vi "Real time state machine - Saccade suppression LED.vi"() -> ()   [LabVIEW 2013]
uses:
  <vilib>/Platform/TimedLoop/XDataNode/timing_clust.ctl
  <vilib>/Platform/TimedLoop/XDataNode/nitl_modes.ctl
  <vilib>/Platform/TimedLoop/XDataNode/wakeup.ctl
  <vilib>/DAQmx/write.llb/DAQmx Write (Digital 1D Bool NChan 1Samp 1Line).vi
  <vilib>/DAQmx/read.llb/DAQmx Read (Analog 1D DBL NChan 1Samp).vi
  <vilib>/DAQmx/write.llb/DAQmx Write (Analog DBL 1Chan 1Samp).vi
  <vilib>/platform/TimedLoop/XDataNode/XDataNode.xnode
  <vilib>/Platform/TimedLoop/XDataNode/XDNodeRunTimeDep.lvlib
panel:
  out "x degree out":dbl
  in  "Saccade min degrees per 3 frames":dbl=5.0
  in  "Saccade max degrees per 3 frames":dbl=15.0
  out "Min":dbl
  out "Sec":dbl=47.16078567504883
  in  "Display length (S)":sgl=10.0
  out "shaft encoder":waveform(sgl)(graph)={"t0"=timestamp(3524542772.3366966 s since 1904-01-01), "dt"=0.02, "Y"=array[500 elements]}
  out "Current state":T1(ring)=enum."VS"
  out "# of rewards":i32
  in  "Automatic reward":bool=TRUE
  out "Lick reward":bool
  out "RT FIFO (DISP)":u32(slide) scale=0.0..50.0
  out "RT FIFO (Log)":u32(slide) scale=0.0..50.0
  out "Digital Waveform Graph":digitalwaveform(graph)={"t0"=timestamp(3524542772.3366966 s since 1904-01-01), "dt"=0.0004, "Y"={"transitions"=[], "data"=array25000x3[75000 elements]}, "error"={"status"=FALSE, "code"=37421928, "source"=""}}
  out "Trial # (State machine)":u32=1
  out "Actual cycle period (uS)":i64=94
  in  "State machine cycle (uS)":i64=200
  in  "Save file to":string="C:\\ni-rt\\LabVIEW Data\\"
  in  "RT FIFO size":u32=50
  in  "VS filter period (uS)":i32=500
  out "Start one trial":bool
  out "Trial Done":bool
  out "error out":errorcluster
  out "Busy":bool
  out "Trial #":i32=1
  out "Save data":bool
  out "LED?":bool
  out "Pulse amp 0":sgl
  out "Pulse amp 1":sgl
  out "Pulse delay":sgl
  out "Pulse width":sgl
  out "Pulse period (ms)":sgl
  out "Pulse #":sgl
  out "Reward period (uS)":u32
  out "Reward start delay (uS)":u32
  out "Water duration (uS)":u32=30000
  out "Water refractory period (uS)":u32=500000
  out "Shock duration (uS)":u32=10000
  out "Shock refractory period (uS)":u32=1000000
  out "Trial timeout (uS)":u32=3000000
  out "Lick threshold (V)":fxp<+,32,16>=1.600006103515625
  out "Track eye":bool=TRUE
  out "Allow shock":bool
  out "Allow timeout":bool
  out "Manually give water":bool
  out "Manually give shock":bool
  out "VS threshold (V)":fxp<+,32,16>=0.5
  out "VS type":string="continuous_flash"
  out "File name":string="Test"
  out "Behavior type":string="fullfield"
  in  "Stop state":bool
  in  "Remote port":u16=9090
  in  "Remote IP_Main":string="192.168.137.10"
  in  "Local port":u16=9091
  in  "Local IP_This computer":string="192.168.137.2"
  out "ABORT":bool
  out "Initial data received":bool
  # "VS"
  # "Behavior"
  # "Trial #"
  # "Received parameters"
  # "Time to wait for reward window"
  # "Elapsed time"
  # "Min"
  # "Sec"
  # "Controls"
  # "Network"
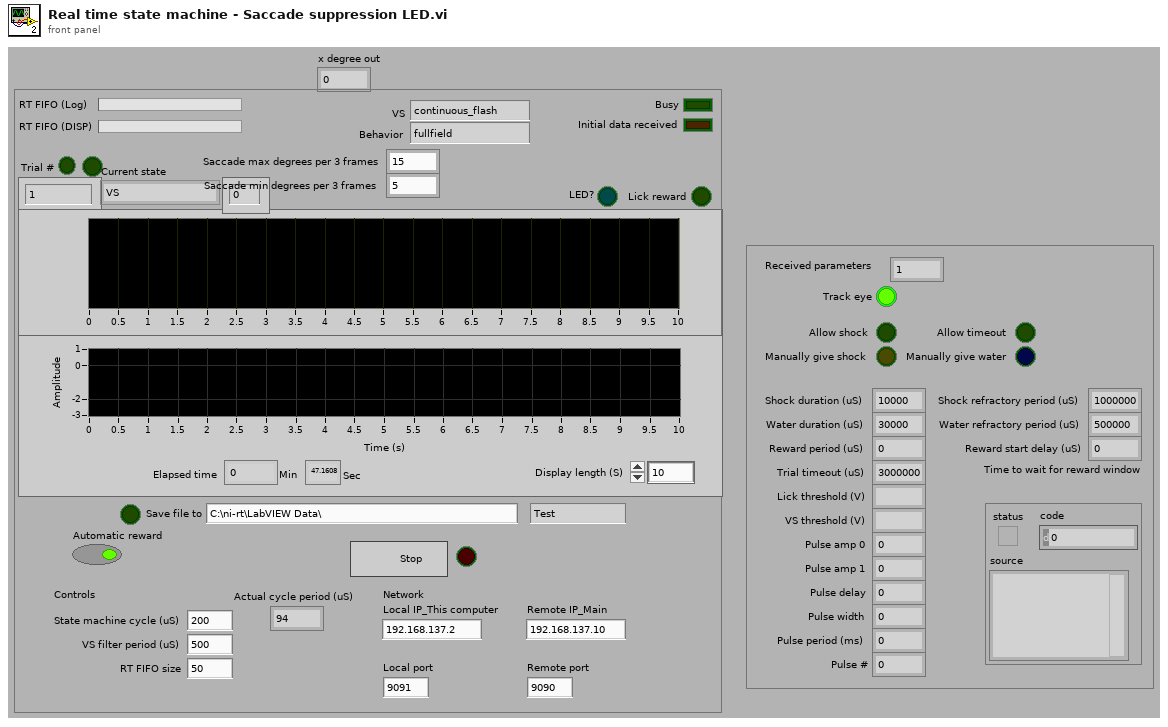
[diagram p1: front panel]
types:
  T1 = enum16{"Idle", "Before VS", "VS", "VS2", "After VS", "Wait for lever press", "Cycle End", "Reward", "Reward Refractory", "Punish", "Punish Refractory", "Exit", "Timeout", "Lick reward"}
  T2 = enum16{"open", "replace", "create", "open or create", "replace or create", "replace or create with confirmation"}
  T3 = typedef "XDNodeRunTimeDep.lvlib/timing_clust.ctl" = cluster{"Expected End [f-1]":u64, "Actual End [f-1]":u64, "Finished Late? [f-1]":bool, "Expected End [i-1]":u64, "Actual End [i-1]":u64, "Finished Late? [i-1]":bool, "Expected Start [i]":u64, "Actual Start [i]":u64, "Expected Start [f]":u64, "Actual Start [f]":u64, "Source Name":string, "Structure Name":string, "Period":i64, "Deadline":i64, "Offset":i64, "Start":i64, "Priority":i32, "Timeout":i32, "Mode":T4, "Wakeup Reason":T5, "Error":errorcluster, "Source Type":string, "Secondary Source Type":string, "Global End Time":u64, "Global Start Time":u64, "Frame Duration":u64, "Iteration Duration":u64, "Assigned CPU":i32, "I/O Scan Engine Mode":u32}
  T4 = typedef "XDNodeRunTimeDep.lvlib/nitl_modes.ctl" = enum32{"No Change", "Process missed periods, maintain original phase", "Discard missed periods, maintain original phase", "Process missed periods, ignore original phase", "Discard missed periods, ignore original phase"}
  T5 = typedef "XDNodeRunTimeDep.lvlib/wakeup.ctl" = enum32{"Normal", "Aborted", "Asynchronous wakeup", "Timing source error", "Timed loop error", "Timeout"}
  T6 = enum16{"big-endian, network order", "native, host order", "little-endian"}
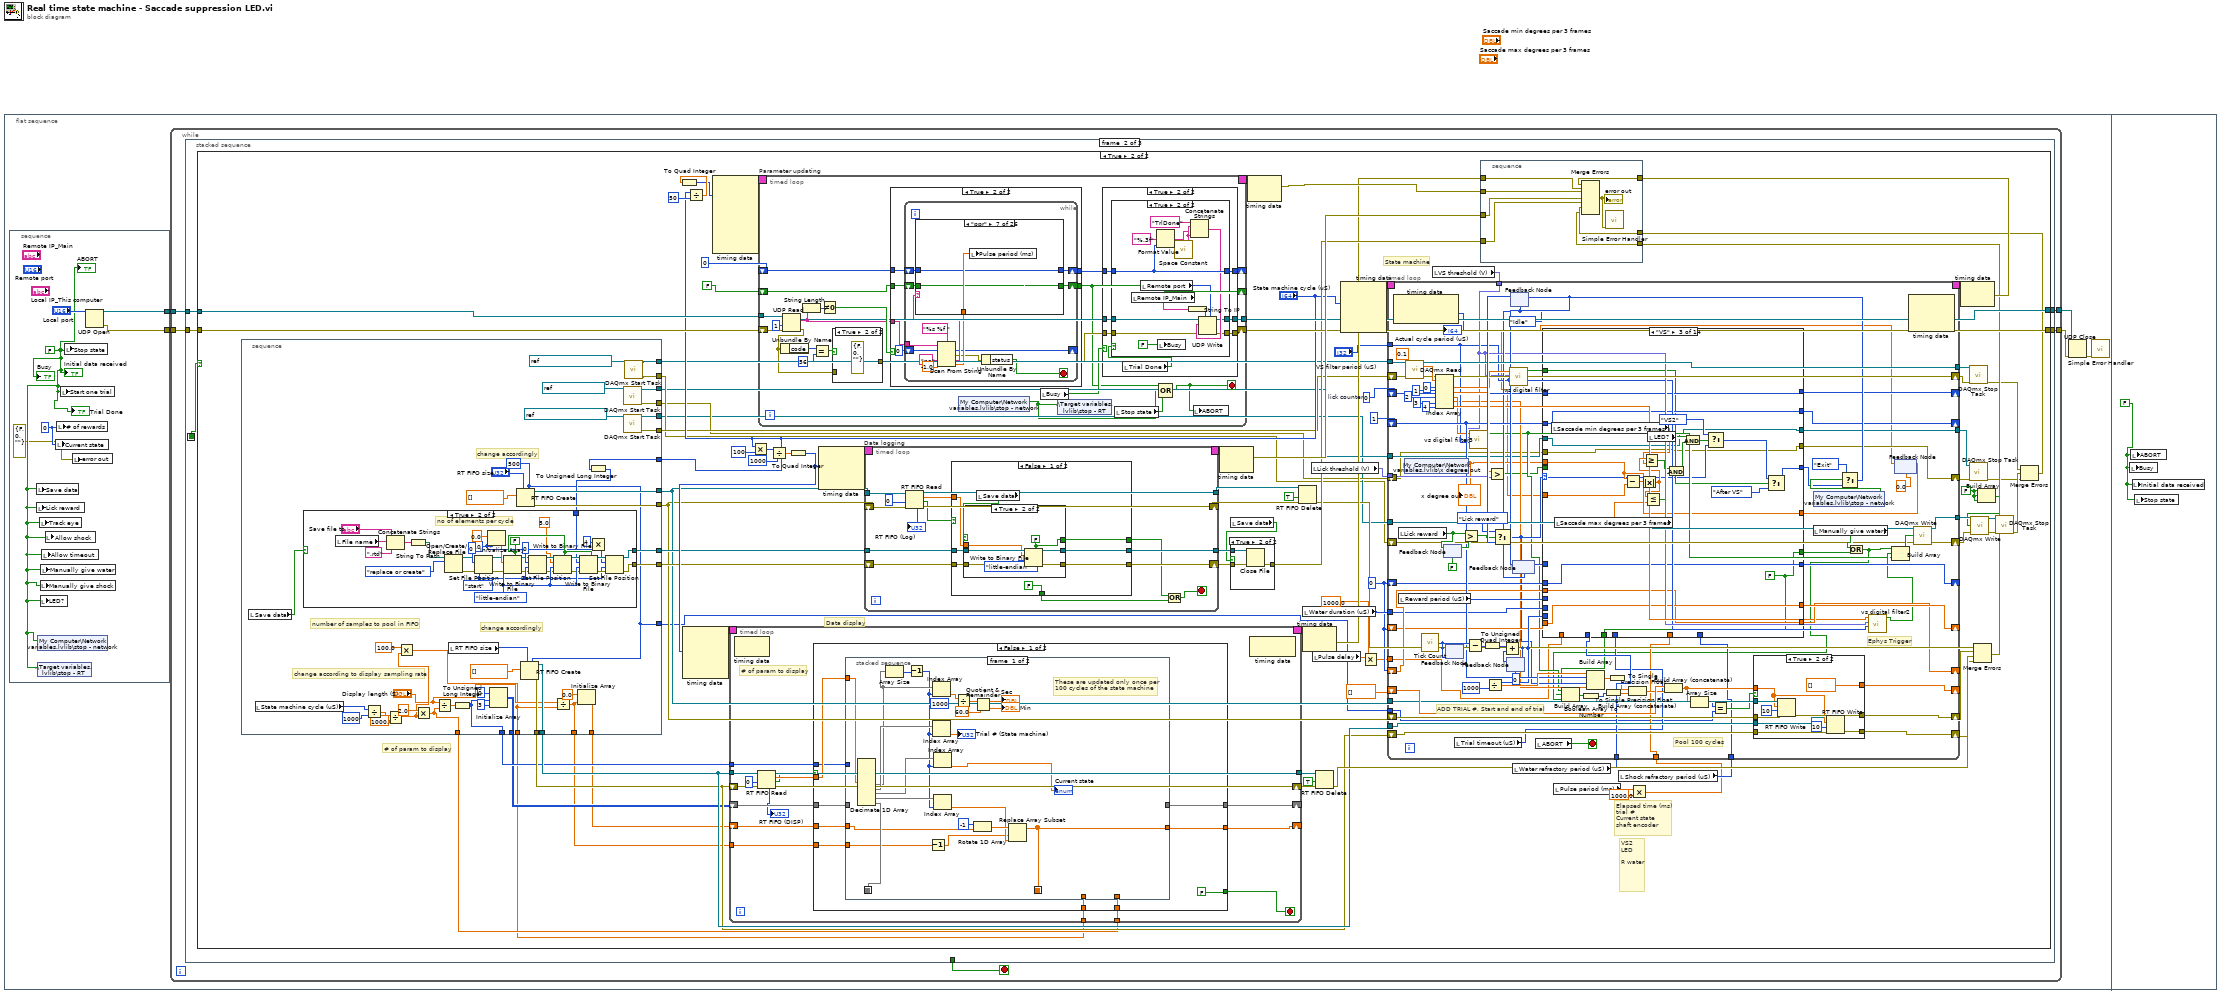
[diagram p0: block diagram]
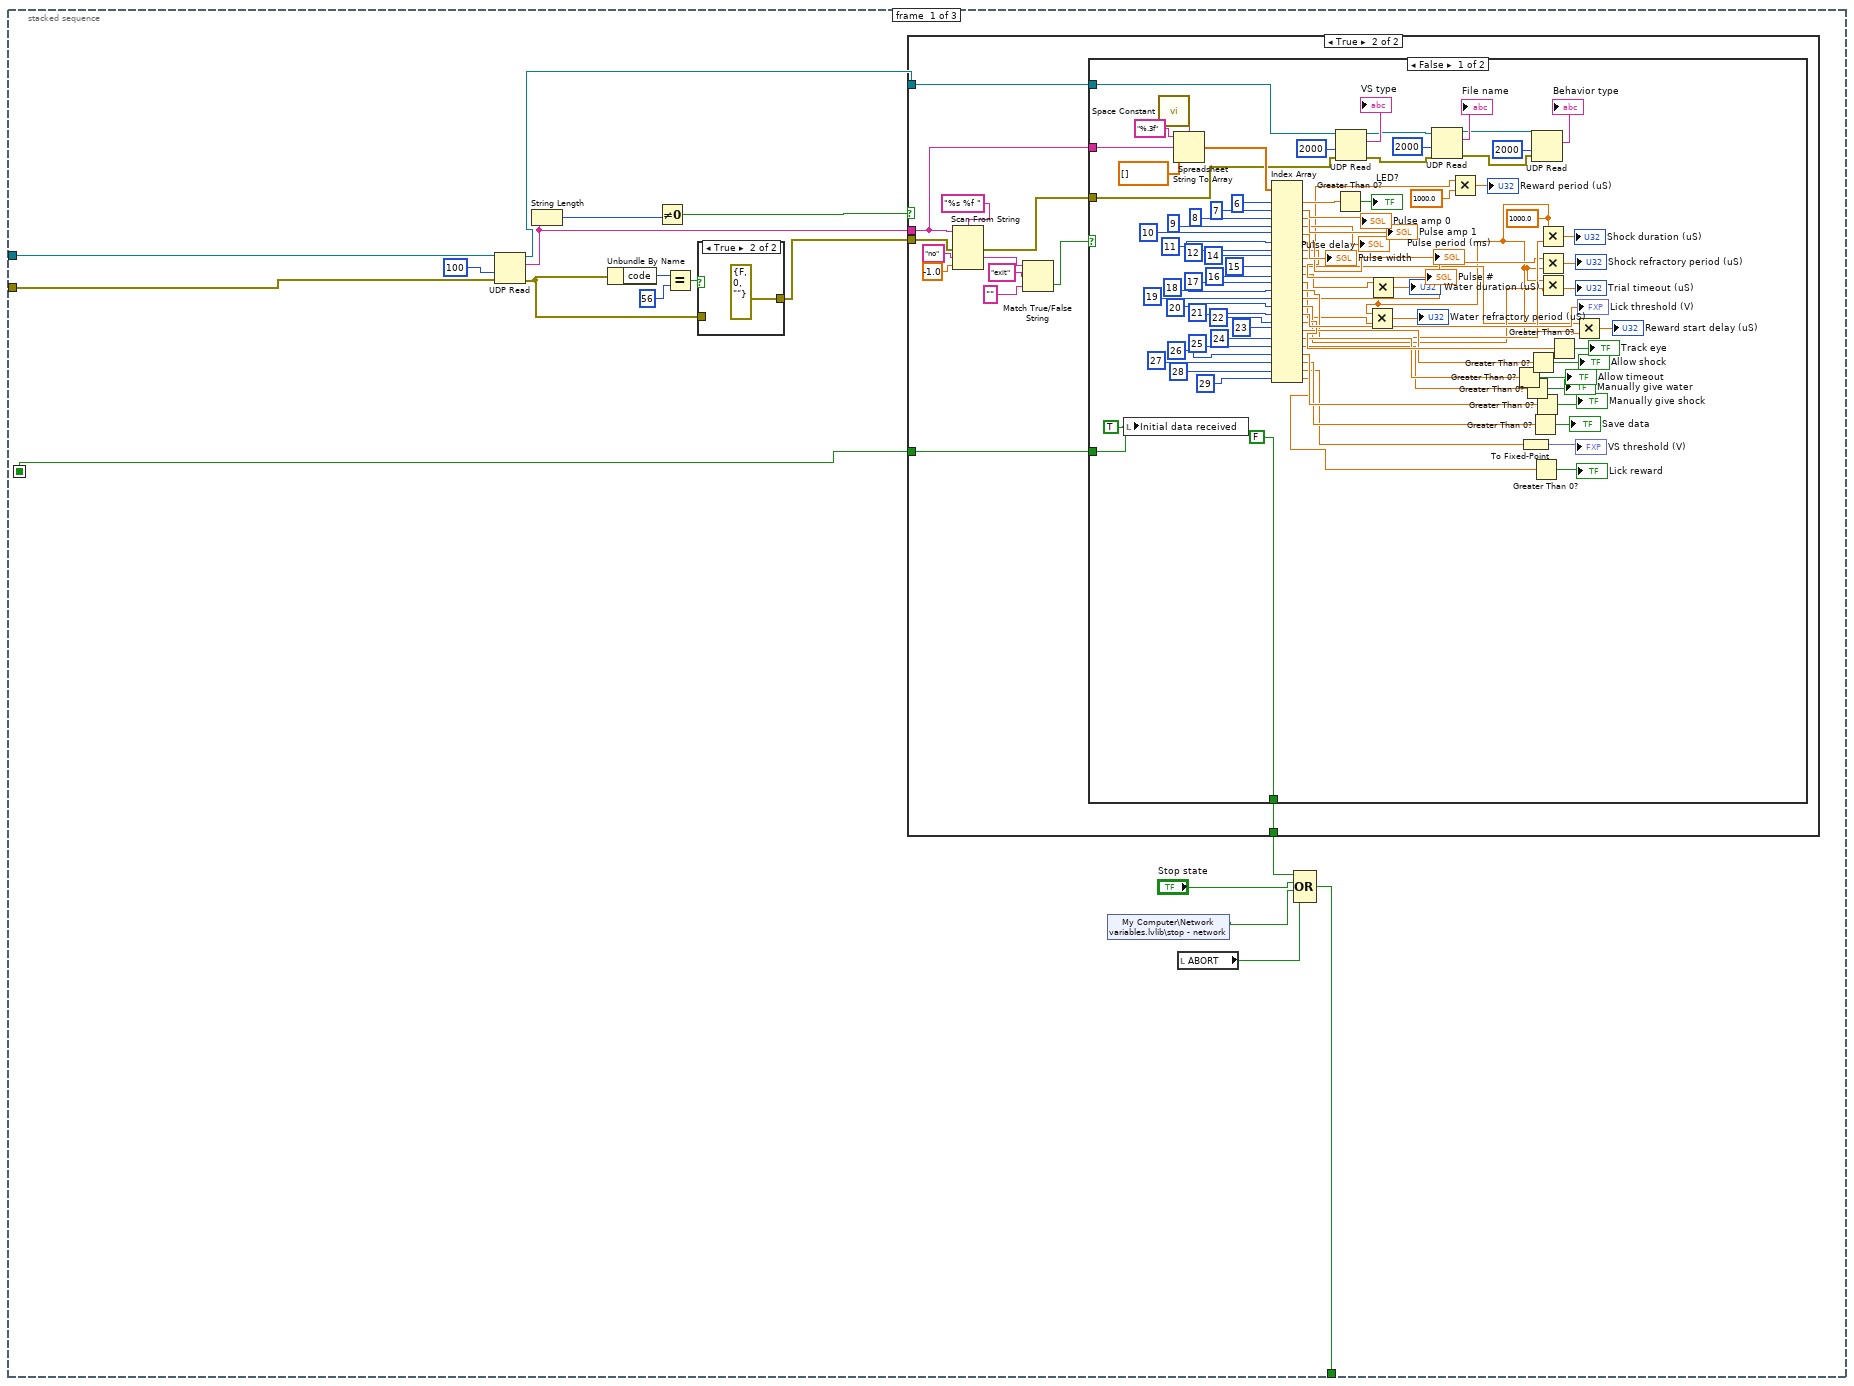
[diagram p2: hidden frame]
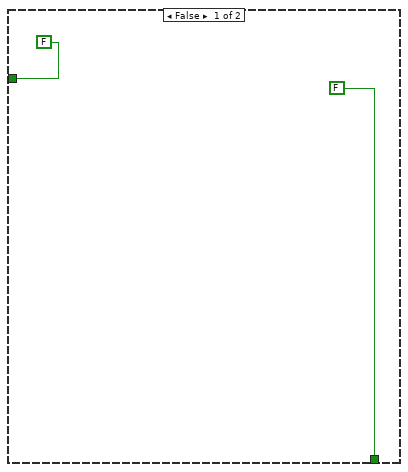
[diagram p3: hidden frame]
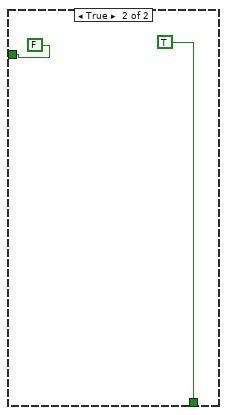
[diagram p4: hidden frame]
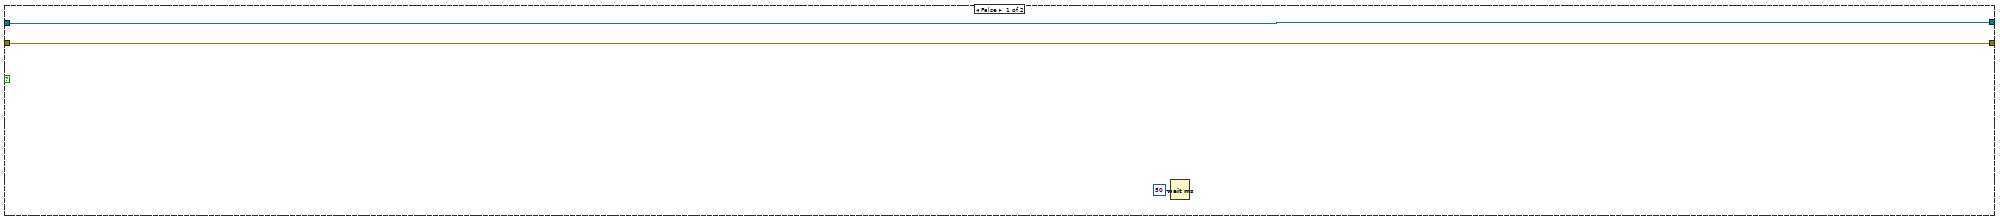
[diagram p6: hidden frame]
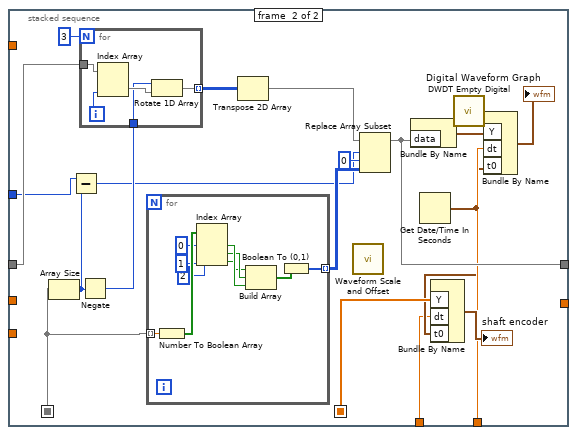
[diagram p9: hidden frame]
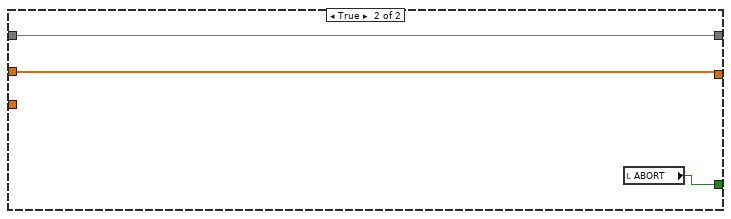
[diagram p10: hidden frame]
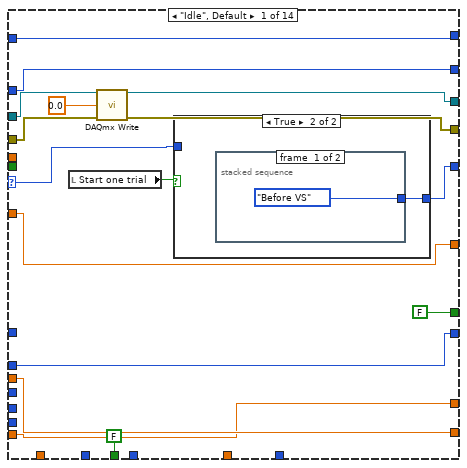
[diagram p11: hidden frame]
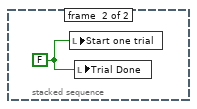
[diagram p13: hidden frame]
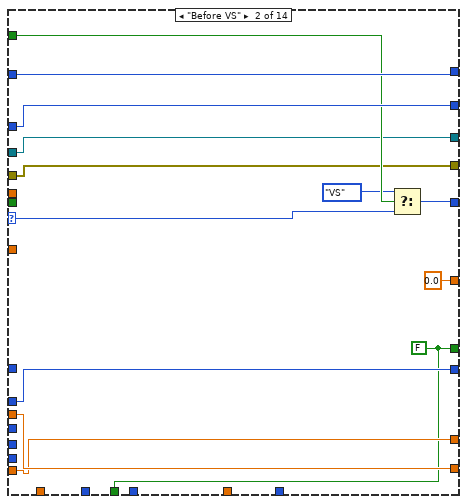
[diagram p14: hidden frame]
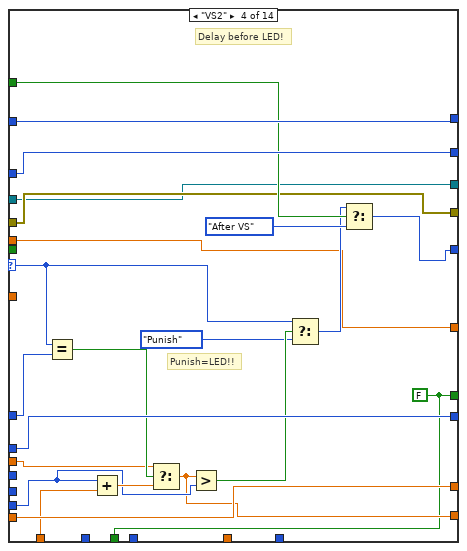
[diagram p15: hidden frame]
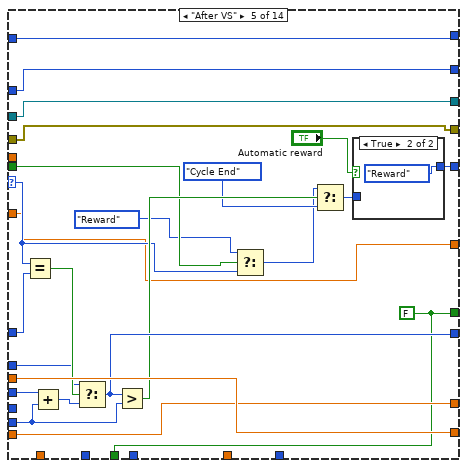
[diagram p16: hidden frame]
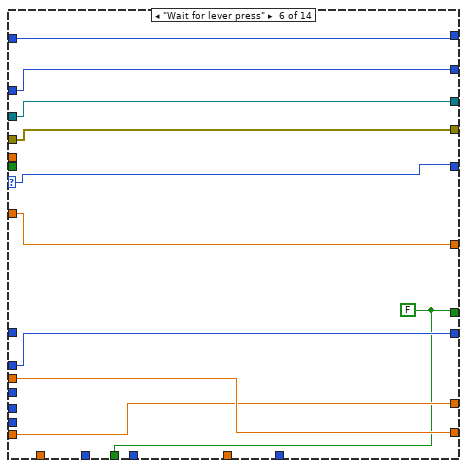
[diagram p18: hidden frame]
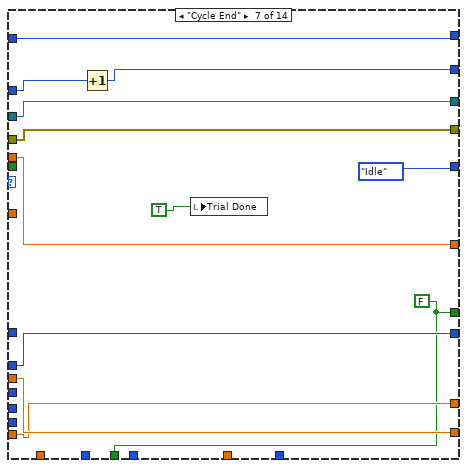
[diagram p19: hidden frame]
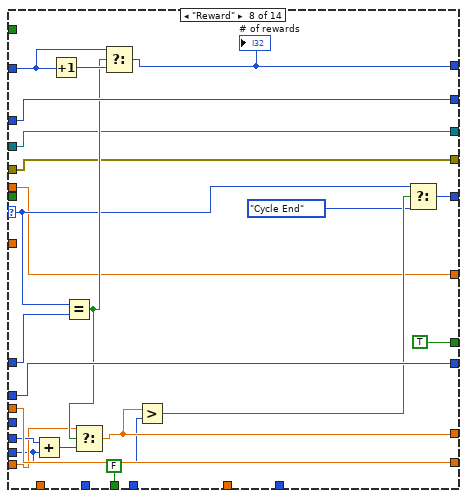
[diagram p20: hidden frame]
diagram:
  n1 = flat-sequence {
    frame #0 {
      n2 = stacked-sequence {
        tunnel: [w1027] -> w5
        tunnel: [w1026] -> w4
        frame #0 {
          w1025 = 0
          w1024 = FALSE
          n3 = local write "Save data"(w1024) -> ()
          n4 = local write "Lick reward"(w1024) -> ()
          n5 = shared-variable "My Computer\\Network variables.lvlib\\stop - network"(w1024) -> ()  [unwired: 1 in, 1 out]
          n6 = shared-variable ".\\Target variables.lvlib\\stop - RT"(w1024) -> ()  [unwired: 1 in, 1 out]
          n7 = local write "Track eye"(w1024) -> ()
          n8 = local write "Manually give shock"(w1024) -> ()
          n9 = local write "LED?"(w1024) -> ()
          n10 = local write "Manually give water"(w1024) -> ()
          n11 = local write "Allow timeout"(w1024) -> ()
          n12 = local write "Allow shock"(w1024) -> ()
          n13 = local write "Current state"(w1025) -> ()
          n14 = local write "# of rewards"(w1025) -> ()
          n15 = local write "Start one trial"(w1024) -> ()
          n16 = local write "Stop state"(w1024) -> ()
          n17 = local write "error out"(errorcluster {"status"=FALSE, "code"=0, "source"=""} ("error out")) -> ()
          n18 = UDP Open(11:"Local port") -> (port=w1027:refnum<k16>, 0:w1026:errorcluster)  [unwired: 4 in, 1 out]
          "ABORT" <- w1024
          "Initial data received" <- w1024
          "Busy" <- w1024
          "Trial Done" <- w1024
        }
      }
      n19 = while {
        tunnel: w5 -> [w10]
        tunnel: w4 -> [w9]
        tunnel: [w8] -> w3
        tunnel: [w7] -> w2
        stop <- w6 stop-if-true
        n20 = stacked-sequence {
          seq-local: [w16 _ _] -> [_ w135 _]
          tunnel: w10 -> [w27 w132 _]
          tunnel: w9 -> [w26 w133 _]
          tunnel: [w15 _ _] -> w6
          tunnel: [_ w134 _] -> w8
          tunnel: [_ w131 _] -> w7
          frame #0 {
            n21 = UDP Read(connection ID=w27, timeout ms (25000)=100, 8:w26) -> (data out=w18:string, error out=w22:errorcluster, 3:w17:refnum<k16>)  [unwired: 1 in, 2 out]
            n22 = String Length(string=w18) -> (length=w21:i32)
            n23 = Unbundle By Name(w22) -> ("code"=w25:i32)
            n24 = Not Equal To 0?(x=w21) -> (x != 0?=w20:bool)
            n25 = Equal?(x=w25, y=56) -> (x = y?=w23:bool)
            n26 = case shown="True" w23 {
              tunnel: w22 -> [w129 _]
              tunnel: [w129 errorcluster {"status"=FALSE, "code"=0, "source"=""} ("error out")] -> w19
              frame False {
              }
              frame True {
              }
            }
            n27 = case shown="True" w20 {
              tunnel: w19 -> [_ w41]
              tunnel: w18 -> [_ w35]
              tunnel: w17 -> [_ w33]
              tunnel: [FALSE w32] -> w14
              tunnel: [FALSE w31] -> w16
              frame False {
              }
              frame True {
                n28 = Scan From String(format string="%s %f ", input string=w35, error in=w41, default 1="no" ("default value 1"), default 2=sgl -1.0 ("default value 1")) -> (error out=w34:errorcluster, output 1=w39:string)  [unwired: 2 in, 2 out]
                n29 = Match True/False String(2:"" ("false string"), 3:"exit" ("true string"), 4:w39) -> (0:w36:bool)  [unwired: 1 out]
                n30 = case shown="False" w36 {
                  tunnel: w35 -> [w123 _]
                  tunnel: w34 -> [w81 _]
                  tunnel: w33 -> [w80 _]
                  tunnel: [FALSE TRUE] -> w32
                  tunnel: [w68 FALSE] -> w31
                  frame False {
                    w49 = sgl 1000.0
                    w68 = TRUE
                    n31 = local write "Initial data received"(w68) -> ()
                    n32 = call <vilib>:"Space Constant.vi"() -> ("String"=w125:string)
                    n33 = Spreadsheet String To Array(delimiter (Tab)=w125, format string="%.3f", spreadsheet string=w123, array type (2D Dbl)=sgl[] []) -> (array=w122:sgl[])
                    n34 = Index Array(array=w122, index #1=6 ("index"), index #2=7 ("index"), index #3=8 ("index"), index #4=9 ("index"), index #5=10 ("index"), index #6=11 ("index"), index #7=12 ("index"), index #8=14 ("index"), index #9=15 ("index"), index #10=16 ("index"), index #11=17 ("index"), index #12=18 ("index"), index #13=19 ("index"), index #14=20 ("index"), index #15=21 ("index"), index #16=22 ("index"), index #17=23 ("index"), index #18=24 ("index"), index #19=25 ("index"), index #20=26 ("index"), index #21=27 ("index"), index #22=28 ("index"), index #23=29 ("index")) -> (element #1=w120:sgl, element #2=→"Pulse amp 0":sgl, element #3=→"Pulse amp 1":sgl, element #4=→"Pulse delay":sgl, element #5=→"Pulse width":sgl, element #6=→"Pulse period (ms)":sgl, element #7=→"Pulse #":sgl, element #8=w64:sgl, element #9=w55:sgl, element #10=w53:sgl, element #11=w51:sgl, element #12=w61:sgl, element #13=w60:sgl, element #14=w57:sgl, element #15=→"Lick threshold (V)":sgl, element #16=w94:sgl, element #17=w91:sgl, element #18=w89:sgl, element #19=w86:sgl, element #20=w84:sgl, element #21=w46:sgl, element #22=w45:sgl, element #23=w44:sgl)
                    n35 = Greater Than 0?(x=w120) -> (x > 0?=→"LED?":bool)
                    n36 = UDP Read(connection ID=w80, timeout ms (25000)=2000, 8:w81) -> (data out=→"VS type":string, error out=w76:errorcluster, 3:w74:refnum<k16>)  [unwired: 1 in, 2 out]
                    n37 = Multiply(x=w49, y=w51) -> (x*y=→"Water refractory period (uS)":sgl)
                    n38 = Multiply(x=w53, y=w49) -> (x*y=→"Water duration (uS)":sgl)
                    n39 = UDP Read(connection ID=w74, timeout ms (25000)=2000, 8:w76) -> (data out=→"File name":string, error out=w72:errorcluster, 3:w71:refnum<k16>)  [unwired: 1 in, 2 out]
                    n40 = Multiply(x=w64, y=sgl 1000.0) -> (x*y=→"Reward period (uS)":sgl)
                    n41 = Greater Than 0?(x=w89) -> (x > 0?=→"Allow timeout":bool)
                    n42 = To Fixed-Point(number=w45) -> (fixed-point=→"VS threshold (V)":fxp<+/-,32,16>)  [unwired: 1 in]
                    n43 = Greater Than 0?(x=w86) -> (x > 0?=→"Manually give water":bool)
                    n44 = Greater Than 0?(x=w91) -> (x > 0?=→"Allow shock":bool)
                    n45 = Greater Than 0?(x=w46) -> (x > 0?=→"Save data":bool)
                    n46 = Greater Than 0?(x=w44) -> (x > 0?=→"Lick reward":bool)
                    n47 = UDP Read(connection ID=w71, timeout ms (25000)=2000, 8:w72) -> (data out=→"Behavior type":string)  [unwired: 1 in, 4 out]
                    n48 = Greater Than 0?(x=w84) -> (x > 0?=→"Manually give shock":bool)
                    n49 = Multiply(x=w49, y=w61) -> (x*y=→"Shock duration (uS)":sgl)
                    n50 = Multiply(x=w60, y=w49) -> (x*y=→"Shock refractory period (uS)":sgl)
                    n51 = Multiply(x=w49, y=w57) -> (x*y=→"Trial timeout (uS)":sgl)
                    n52 = Greater Than 0?(x=w94) -> (x > 0?=→"Track eye":bool)
                    n53 = Multiply(x=w55, y=w49) -> (x*y=→"Reward start delay (uS)":sgl)
                  }
                  frame True {
                  }
                }
              }
            }
            n54 = shared-variable "My Computer\\Network variables.lvlib\\stop - network"() -> (w11:bool)  [unwired: 1 in, 1 out]
            n55 = local read "ABORT"() -> (w12:bool)
            n56 = Compound Arithmetic op=OR(w14, "Stop state", w11, w12) -> (w15:bool)
          }
          frame #1 {
            n57 = case shown="True" w135 {
              tunnel: w133 -> [w138 w221]
              tunnel: [w138 w213] -> w134
              tunnel: w132 -> [w137 w220]
              tunnel: [w137 w212] -> w131
              frame False {
                n58 = Wait (ms)(milliseconds to wait=u32 50) -> ()  [unwired: 1 out]
              }
              frame True {
                w165 = FALSE
                w201 = 0  # lick counter
                w158 = 0
                # "VS2\nLED\n\nR water"
                # "# of param to display"
                # "Data display"
                # "Elapsed time (ms)\ntrial #\nCurrent state\nshaft encoder"
                # "State machine"
                n59 = stacked-sequence {
                  tunnel: [w273] -> w186
                  tunnel: [w272] -> w185
                  tunnel: [w269] -> w184
                  tunnel: [w268] -> w183
                  tunnel: [w254] -> w166
                  tunnel: [w249] -> w182
                  tunnel: [w260] -> w181
                  tunnel: "State machine cycle (uS)" -> [w253]
                  tunnel: [w257] -> w179
                  tunnel: [w256] -> w178
                  tunnel: [w251] -> w157
                  tunnel: [w248] -> w156
                  tunnel: [w244] -> w155
                  tunnel: [w243] -> w154
                  tunnel: [w241] -> w144
                  tunnel: [w240] -> w143
                  tunnel: [w238] -> w142
                  tunnel: [w237] -> w141
                  tunnel: [w235] -> w140
                  tunnel: [w234] -> w139
                  frame #0 {
                    w251 = u32 500 ("elements in array (1)")
                    # "number of samples to pool in FIFO"
                    # "change according to display sampling rate"
                    # "change accordingly"
                    # "change accordingly"
                    n60 = local read "Save data"() -> (w274:bool)
                    n61 = local read "State machine cycle (uS)"() -> (w261:i64)
                    n62 = Divide(x=w261, y=u32 1000) -> (x/y=w263:dbl)
                    n63 = Divide(x=w263, y=1000.0) -> (x/y=w246:dbl)
                    n64 = Multiply(x=100.0, y=w246) -> (x*y=w244:dbl)
                    n65 = Multiply(x=2.0, y=w246) -> (x*y=w254:dbl)
                    n66 = Divide(x="Display length (S)", y=w254) -> (x/y=w266:dbl)
                    n67 = local read "RT FIFO size"() -> (w271:u32)
                    n68 = To Unsigned Long Integer(number=w266) -> (unsigned 32bit integer=w249:u32)
                    n69 = Initialize Array(u8 0 ("element"), w249, 3 ("dimension size")) -> (w260:u8[][])
                    n70 = RT FIFO Create(1:sgl[] [], 4:"RT FIFO size", 6:w251) -> (8:w257:refnum<k33>, 11:w256:errorcluster)  [unwired: 5 in, 1 out]
                    n71 = RT FIFO Create(1:sgl[] [], 4:w271, 6:w251) -> (8:w269:refnum<k33>, 11:w268:errorcluster)  [unwired: 5 in, 1 out]
                    n72 = Divide(x="Display length (S)", y=w244) -> (x/y=w243:dbl)
                    n73 = Initialize Array(sgl 0.0 ("element"), w243) -> (w248:sgl[])
                    n74 = To Unsigned Long Integer(number=w253) -> (unsigned 32bit integer=w252:u32)
                    n75 = case shown="True" w274 {
                      tunnel: [_ w278] -> w273
                      tunnel: [_ w277] -> w272
                      tunnel: w252 -> [_ w276]
                      frame False {
                      }
                      frame True {
                        w299 = FALSE
                        w292 = 10 ("dimension size")
                        w300 = T6."little-endian" ("byte order (0:big-endian, network order)")
                        w291 = enum16{"start", "end", "current"}."start" ("from (0:start)")
                        # "no of elements per cycle"
                        n76 = local read "File name"() -> (w302:string)
                        n77 = Concatenate Strings("Save file to", w302, ".rtd" ("string")) -> (w305:string)
                        n78 = String To Path(string=w305) -> (path=w306:path)
                        n79 = Open/Create/Replace File(file path (use dialog)=w306, operation (0:open)=T2."replace or create") -> (refnum out=w279:refnum<file>, error out=w280:errorcluster)  [unwired: 4 in, 1 out]
                        n80 = Set File Position(offset (in bytes) (0)=i64 0, refnum=w279, from (0:start)=w291, error in=w280) -> (refnum out=w282:refnum<file>, error out=w283:errorcluster)
                        n81 = Initialize Array(sgl 0.0 ("element"), w292) -> (w285:sgl[])
                        n82 = Write to Binary File(file (use dialog)=w282, data=w285, error in=w283, 5:w299, 9:w300) -> (refnum out=w287:refnum<file>, error out=w286:errorcluster)  [unwired: 1 in, 1 out]
                        n83 = Set File Position(offset (in bytes) (0)=i64 0, refnum=w287, from (0:start)=w291, error in=w286) -> (refnum out=w289:refnum<file>, error out=w290:errorcluster)
                        n84 = Write to Binary File(file (use dialog)=w289, data=sgl 5.0, error in=w290, 5:w299, 9:w300) -> (refnum out=w297:refnum<file>, error out=w295:errorcluster)  [unwired: 1 in, 1 out]
                        n85 = Write to Binary File(file (use dialog)=w297, data=w276, error in=w295, 5:w299, 9:w300) -> (refnum out=w298:refnum<file>, error out=w296:errorcluster)  [unwired: 1 in, 1 out]
                        n86 = Multiply(x=4, y=w292) -> (x*y=w294:i32)
                        n87 = Set File Position(offset (in bytes) (0)=w294, refnum=w298, from (0:start)=w291, error in=w296) -> (refnum out=w277:refnum<file>, error out=w278:errorcluster)
                      }
                    }
                    n88 = call <vilib>:"DAQmx Start Task.vi"("task/channels in"=refnum<k21> "LED analog out" ("DAQmx Task Name")) -> ("task out"=w238:refnum<k21>, "error out"=w237:errorcluster)  [unwired: 13 in]
                    n89 = call <vilib>:"DAQmx Start Task.vi"("task/channels in"=refnum<k21> "Digital_write_saccade" ("DAQmx Task Name")) -> ("task out"=w235:refnum<k21>, "error out"=w234:errorcluster)  [unwired: 13 in]
                    n90 = call <vilib>:"DAQmx Start Task.vi"("task/channels in"=refnum<k21> "Analog_read_saccade" ("DAQmx Task Name")) -> ("task out"=w241:refnum<k21>, "error out"=w240:errorcluster)  [unwired: 13 in]
                  }
                }
                n91 = Divide(x="State machine cycle (uS)", y=i64 50) -> (x/y=w191:dbl)
                n92 = To Quad Integer(1:w191) -> (0:w190:i64)
                n93 = node-c288 ("Input Node")(w190) -> (w229:T3)  [unwired: 6 in]
                n94 = Multiply(x="State machine cycle (uS)", y=u32 100) -> (x*y=w194:i64)
                n95 = timed-loop "Parameter updating" {
                  timing: w229 -> [_]
                  timing-out: [_] -> w228
                  tunnel: w220 -> [w860]
                  shift-right: [w845] -> w213
                  shift-left: w221 -> [w861]
                  shift-right: [w848] -> _
                  shift-left: 0 -> [w851]
                  tunnel: [w844] -> w212
                  shift-right: [w842] -> _
                  shift-left: FALSE -> [w852]
                  stop <- w843 stop-if-true
                  n96 = UDP Read(connection ID=w860, timeout ms (25000)=1, 8:w861) -> (data out=w853:string, error out=w856:errorcluster, 3:w846:refnum<k16>)  [unwired: 1 in, 2 out]
                  n97 = Unbundle By Name(w856) -> ("code"=w859:i32)
                  n98 = String Length(string=w853) -> (length=w855:i32)
                  n99 = Equal?(x=w859, y=56) -> (x = y?=w857:bool)
                  n100 = Not Equal To 0?(x=w855) -> (x != 0?=w854:bool)
                  n101 = case shown="True" w857 {
                    tunnel: w856 -> [w1013 _]
                    tunnel: [w1013 errorcluster {"status"=FALSE, "code"=0, "source"=""} ("error out")] -> w847
                    frame False {
                    }
                    frame True {
                    }
                  }
                  n102 = case shown="True" w854 {
                    tunnel: w853 -> [_ w896]
                    tunnel: w852 -> [w889 w895]
                    tunnel: w851 -> [w890 w894]
                    tunnel: [w890 w893] -> w849
                    tunnel: [w889 w892] -> w842
                    frame False {
                    }
                    frame True {
                      n103 = while {
                        tunnel: w896 -> [w908]
                        shift-right: [w904] -> w892
                        shift-left: w895 -> [w905]
                        shift-right: [w903] -> w893
                        shift-left: w894 -> [w902]
                        shift-right: [w898] -> _
                        shift-left: u32 0 -> [w899]
                        stop <- w900 stop-if-true
                        n104 = Scan From String(format string="%s %f ", input string=w908, initial scan location=w899, default 1="no" ("default value 1"), default 2=-1.0 ("default value 2")) -> (offset past scan=w898:u32, error out=w901:errorcluster, output 1=w907:string, output 2=w906:dbl)  [unwired: 1 in, 1 out]
                        n105 = case shown="\"ppr\"" w907 {
                          tunnel: w906 -> [_ w915 w919 w922 w925 w928 w931 w934 w936 w940 w945 w951 w956 w961 w966 w972 w975 w979 w984 w987 w991 w995 w998 w1002 _ _]
                          tunnel: w905 -> [w912 w913 w917 w920 w923 w926 w929 w932 w938 w943 w948 w953 w958 w963 w968 w970 w973 w977 w981 w985 w989 w993 w999 w1003 w1006 w1011]
                          tunnel: [w912 w913 w917 w920 w923 w926 w929 w932 w938 w943 w948 w953 w958 w963 w968 w970 w973 w977 w981 w985 w989 w993 w999 w1003 w1006 w1010] -> w904
                          tunnel: [w911 w914 w918 w921 w924 w927 w930 w933 w939 w944 w949 w954 w959 w964 w969 w971 w974 w978 w982 w986 w990 w994 w1000 w1004 w1007 w1009] -> w903
                          tunnel: w902 -> [w911 w914 w918 w921 w924 w927 w930 w933 w939 w944 w949 w954 w959 w964 w969 w971 w974 w978 w982 w986 w990 w994 w1000 w1004 w1008 w1009]
                          frame "no", Default {
                          }
                          frame "led" {
                            n106 = Greater Than 0?(x=w915) -> (x > 0?=w916:bool)
                            n107 = local write "LED?"(w916) -> ()
                          }
                          frame "pai" {
                            n108 = local write "Pulse amp 0"(w919) -> ()
                          }
                          frame "paf" {
                            n109 = local write "Pulse amp 1"(w922) -> ()
                          }
                          frame "pdl" {
                            n110 = local write "Pulse delay"(w925) -> ()
                          }
                          frame "pwd" {
                            n111 = local write "Pulse width"(w928) -> ()
                          }
                          frame "ppr" {
                            n112 = local write "Pulse period (ms)"(w931) -> ()
                          }
                          frame "pnm" {
                            n113 = local write "Pulse #"(w934) -> ()
                          }
                          frame "rwp" {
                            n114 = Multiply(x=1000.0, y=w936) -> (x*y=w935:dbl)
                            n115 = local write "Reward period (uS)"(w935) -> ()
                          }
                          frame "rwd" {
                            n116 = Multiply(x=1000.0, y=w940) -> (x*y=w941:dbl)
                            n117 = local write "Reward start delay (uS)"(w941) -> ()
                          }
                          frame "wdr" {
                            n118 = Multiply(x=1000.0, y=w945) -> (x*y=w946:dbl)
                            n119 = local write "Water duration (uS)"(w946) -> ()
                          }
                          frame "wre" {
                            n120 = Multiply(x=1000.0, y=w951) -> (x*y=w950:dbl)
                            n121 = local write "Water refractory period (uS)"(w950) -> ()
                          }
                          frame "shd" {
                            n122 = Multiply(x=1000.0, y=w956) -> (x*y=w955:dbl)
                            n123 = local write "Shock duration (uS)"(w955) -> ()
                          }
                          frame "shr" {
                            n124 = Multiply(x=1000.0, y=w961) -> (x*y=w960:dbl)
                            n125 = local write "Shock refractory period (uS)"(w960) -> ()
                          }
                          frame "tto" {
                            n126 = Multiply(x=1000.0, y=w966) -> (x*y=w965:dbl)
                            n127 = local write "Trial timeout (uS)"(w965) -> ()
                          }
                          frame "lkt" {
                            n128 = local write "Lick threshold (V)"(w972) -> ()
                          }
                          frame "etk" {
                            n129 = Greater Than 0?(x=w975) -> (x > 0?=w976:bool)
                            n130 = local write "Track eye"(w976) -> ()
                          }
                          frame "ash" {
                            n131 = Greater Than 0?(x=w979) -> (x > 0?=w980:bool)
                            n132 = local write "Allow shock"(w980) -> ()
                          }
                          frame "ato" {
                            n133 = Greater Than 0?(x=w984) -> (x > 0?=w983:bool)
                            n134 = local write "Allow timeout"(w983) -> ()
                          }
                          frame "gwt" {
                            n135 = Greater Than 0?(x=w987) -> (x > 0?=w988:bool)
                            n136 = local write "Manually give water"(w988) -> ()
                          }
                          frame "gsh" {
                            n137 = Greater Than 0?(x=w991) -> (x > 0?=w992:bool)
                            n138 = local write "Manually give shock"(w992) -> ()
                          }
                          frame "sav" {
                            n139 = Greater Than 0?(x=w995) -> (x > 0?=w996:bool)
                            n140 = local write "Save data"(w996) -> ()
                          }
                          frame "vsh" {
                            n141 = To Fixed-Point(number=w998) -> (fixed-point=w997:fxp<+/-,32,16>)  [unwired: 1 in]
                            n142 = local write "VS threshold (V)"(w997) -> ()
                          }
                          frame "rew" {
                            n143 = Greater Than 0?(x=w1002) -> (x > 0?=w1001:bool)
                            n144 = local write "Lick reward"(w1001) -> ()
                          }
                          frame "start" {
                            w1005 = TRUE
                            n145 = Increment(x=w1008) -> (x+1=w1007:i32)
                            "Trial #" <- w1007
                            n146 = local write "Busy"(w1005) -> ()
                            "Start one trial" <- w1005
                          }
                          frame "stop" {
                            n147 = Or(x=w1011, y=TRUE) -> (x .or. y?=w1010:bool)
                          }
                        }
                        n148 = Unbundle By Name(w901) -> ("status"=w900:bool)
                      }
                    }
                  }
                  n149 = shared-variable "My Computer\\Network variables.lvlib\\stop - network"() -> (w840:bool)  [unwired: 1 in, 1 out]
                  n150 = local read "Busy"() -> (w850:bool)
                  n151 = shared-variable ".\\Target variables.lvlib\\stop - RT"(w840) -> ()  [unwired: 1 in, 1 out]
                  n152 = case shown="True" w850 {
                    tunnel: w849 -> [w864 w870]
                    tunnel: [w864 w869] -> w848
                    tunnel: w847 -> [w862 w868]
                    tunnel: w846 -> [w863 w867]
                    tunnel: [w862 w866] -> w845
                    tunnel: [w863 w865] -> w844
                    frame False {
                    }
                    frame True {
                      n153 = local read "Trial Done"() -> (w871:bool)
                      n154 = case shown="True" w871 {
                        tunnel: [w874 w882] -> w869
                        tunnel: w870 -> [w874 w882]
                        tunnel: w868 -> [w873 w879]
                        tunnel: w867 -> [w872 w878]
                        tunnel: [w873 w876] -> w866
                        tunnel: [w872 w875] -> w865
                        frame False {
                        }
                        frame True {
                          n155 = local read "Remote IP_Main"() -> (w887:string)
                          n156 = local read "Remote port"() -> (w886:u16)
                          n157 = Format Value(format string="%.3f", value (0)=w882) -> (output string=w881:string)  [unwired: 1 in]
                          n158 = local write "Busy"(FALSE) -> ()
                          n159 = call <vilib>:"Space Constant.vi"() -> ("String"=w884:string)
                          n160 = String To IP(1:w887) -> (0:w888:u32)
                          n161 = Concatenate Strings("TrlDone" ("data in"), w884, w881, w884) -> (w880:string)
                          n162 = UDP Write(address=w888, port or service name=w886, connection ID=w878, data in=w880, 8:w879) -> (error out=w876:errorcluster, 3:w875:refnum<k16>)  [unwired: 1 in]
                        }
                      }
                    }
                  }
                  n163 = local read "Stop state"() -> (w841:bool)
                  n164 = Compound Arithmetic op=OR(w842, w840, w841) -> (w843:bool)
                  n165 = local write "ABORT"(w843) -> ()
                }
                n166 = Divide(x=w194, y=u32 1000) -> (x/y=w189:dbl)
                n167 = To Quad Integer(1:w189) -> (0:w188:i64)
                n168 = node-c288(w188) -> (w215:T3)  [unwired: 3 in]
                n169 = timed-loop {
                  timing: w215 -> [_]
                  timing-out: [_] -> w214
                  shift-right: [w320] -> w199
                  shift-left: w183 -> [w321]
                  tunnel: w184 -> [w323]
                  tunnel: [w322] -> w200
                  tunnel: w182 -> [w315]
                  shift-right: [w314] -> _
                  shift-left: w181 -> [w316]
                  tunnel: w166 -> [w313]
                  shift-right: [w309] -> _
                  shift-left: w156 -> [w310]
                  tunnel: w155 -> [w308]
                  tunnel: w154 -> [w307]
                  stop <- w311 stop-if-true
                  # "# of param to display"
                  n170 = node-c288() -> ()  [unwired: 1 in, 1 out]
                  n171 = RT FIFO Read(0:w323, 2:0 ("timeout in ms (0)"), 3:w321) -> (7:→"RT FIFO (DISP)":u32, 8:w322:refnum<k33>, 9:w318:sgl[], 10:w317:bool, 11:w320:errorcluster)  [unwired: 1 in]
                  n172 = case shown="False" w317 {
                    tunnel: w318 -> [w333 _]
                    tunnel: w316 -> [w332 w394]
                    tunnel: w315 -> [w331 _]
                    tunnel: [w330 w394] -> w314
                    tunnel: w313 -> [w329 _]
                    tunnel: [FALSE w393] -> w311
                    tunnel: w310 -> [w327 w392]
                    tunnel: [w326 w392] -> w309
                    tunnel: w308 -> [w325 _]
                    tunnel: w307 -> [w324 _]
                    frame False {
                      n173 = stacked-sequence {
                        seq-local: [w343 _] -> [_ w373]
                        seq-local: [w335 _] -> [_ w359]
                        tunnel: w333 -> [w356 _]
                        tunnel: w332 -> [_ w375]
                        tunnel: w331 -> [_ w368]
                        tunnel: [_ w365] -> w330
                        tunnel: w329 -> [_ w360]
                        tunnel: w327 -> [w340 _]
                        tunnel: [w335 _] -> w326
                        tunnel: w325 -> [_ w357]
                        tunnel: w324 -> [w334 _]
                        frame #0 {
                          # "These are updated only once per \n100 cycles of the state machine"
                          n174 = Decimate 1D Array(w356) -> (w345:sgl[], w346:sgl[], w347:sgl[], w342:sgl[], w343:sgl[])  [unwired: 5 out]
                          n175 = Array Size(array=w345) -> (size(s)=w355:i32)
                          n176 = Decrement(x=w355) -> (x-1=w341:i32)
                          n177 = Decrement(x=w334) -> (x-1=w336:dbl)
                          n178 = Index Array(array=w345, index=w341) -> (element=w354:sgl)
                          n179 = Index Array(array=w346, index=w341) -> (element=→"Trial # (State machine)":sgl)
                          n180 = Index Array(array=w347, index=w341) -> (element=→"Current state":sgl)
                          n181 = Index Array(array=w342, index=w341) -> (element=w338:sgl)
                          n182 = Divide(x=w354, y=u32 1000) -> (x/y=w352:sgl)
                          n183 = Rotate 1D Array(1:w340, 2:-1 ("n")) -> (0:w339:sgl[])
                          n184 = Quotient & Remainder(x=w352, y=60.0) -> (x-y*floor(x/y)=→"Sec":dbl, floor(x/y)=→"Min":dbl)
                          n185 = Replace Array Subset(array=w339, new element=w338, index=w336) -> (w335:sgl[])
                        }
                        frame #1 {
                          n186 = Array Size(array=w373) -> (size(s)=w367:i32)
                          n187 = Subtract(x=w368, y=w367) -> (x-y=w366:u32)
                          n188 = Negate(x=w367) -> (-x=w374:i32)
                          n189 = for {
                            N: 3 -> [_]
                            tunnel: w375 -> [w391]
                            tunnel: w374 -> [w388]
                            tunnel: [w387] -> w371 mode=indexing
                            i -> [w390]
                            n190 = Index Array(array=w391, index (col)=w390) -> (element=w389:u8[])  [unwired: 1 in]
                            n191 = Rotate 1D Array(1:w389, 2:w388) -> (0:w387:u8[])
                          }
                          n192 = for {
                            tunnel: w373 -> [w386] mode=indexing
                            tunnel: [w380] -> w372 mode=indexing
                            n193 = Number To Boolean Array(number=w386) -> (Boolean array=w385:bool[])
                            n194 = Index Array(array=w385, index #1=0 ("index"), index #2=1 ("index"), index #3=2 ("index")) -> (element #1=w379:bool, element #2=w378:bool, element #3=w377:bool)
                            n195 = Build Array(w377, w378, w379) -> (w381:bool[])
                            n196 = Boolean To (0,1)(Boolean=w381) -> (0, 1=w380:i16[])
                          }
                          n197 = Transpose 2D Array(2D array=w371) -> (transposed array=w370:u8[][])
                          n198 = call <vilib>:"Waveform Scale and Offset.vi"() -> ()  [unwired: 10 in, 2 out]
                          n199 = Replace Array Subset(array=w370, new element=w372, index (row)=w366, index (col)=0 ("disabled index (col)")) -> (w365:u8[][])
                          n200 = Bundle By Name("data"=w365) -> (w364:digitaldata)  [unwired: 1 in]
                          n201 = Get Date/Time In Seconds() -> (seconds since 1Jan1904=w358:timestamp)
                          n202 = Bundle By Name("Y"=w359, "dt"=w357, "t0"=w358) -> (→"shaft encoder":waveform(sgl))  [unwired: 1 in]
                          n203 = call <vilib>:"DWDT Empty Digital.vi"() -> ("digital waveform out"=w363:digitalwaveform)  [unwired: 5 in]
                          n204 = Bundle By Name(cluster=w363, "Y"=w364, "dt"=w360, "t0"=w358) -> (→"Digital Waveform Graph":digitalwaveform)
                        }
                      }
                    }
                    frame True {
                      n205 = local read "ABORT"() -> (w393:bool)
                    }
                  }
                  n206 = node-c288() -> ()  [unwired: 1 in, 1 out]
                }
                n207 = node-c288 ("Input Node")(w188) -> (w227:T3)  [unwired: 2 in]
                n208 = timed-loop "Data logging" {
                  timing: w227 -> [_]
                  timing-out: [_] -> w226
                  tunnel: [w809] -> w222
                  tunnel: w185 -> [w807]
                  tunnel: w179 -> [w804]
                  shift-right: [w803] -> w204
                  shift-left: w178 -> [w805]
                  tunnel: [w801] -> w202
                  shift-right: [w808] -> w223
                  shift-left: w186 -> [w806]
                  stop <- w797 stop-if-true
                  n209 = RT FIFO Read(0:w804, 2:0 ("timeout in ms (0)"), 3:w805) -> (7:→"RT FIFO (Log)":u32, 8:w801:refnum<k33>, 9:w799:sgl[], 10:w800:bool, 11:w803:errorcluster)  [unwired: 1 in]
                  n210 = case shown="False" w800 {
                    tunnel: [w817 w830] -> w809
                    tunnel: [w816 w831] -> w808
                    tunnel: w807 -> [w815 w830]
                    tunnel: w806 -> [w814 w831]
                    tunnel: w799 -> [w812 _]
                    tunnel: [FALSE w828] -> w795
                    tunnel: [w810 FALSE] -> w796
                    frame False {
                      n211 = local read "Save data"() -> (w813:bool)
                      n212 = case shown="True" w813 {
                        tunnel: [w820 w827] -> w817
                        tunnel: [w819 w826] -> w816
                        tunnel: w815 -> [w820 w825]
                        tunnel: w814 -> [w819 w824]
                        tunnel: w812 -> [_ w823]
                        tunnel: [w818 w821] -> w810
                        frame False {
                          n213 = local read "ABORT"() -> (w818:bool)
                        }
                        frame True {
                          w821 = FALSE
                          n214 = Write to Binary File(file (use dialog)=w825, data=w823, error in=w824, 5:w821, 9:T6."little-endian" ("byte order (0:big-endian, network order)")) -> (refnum out=w827:refnum<file>, error out=w826:errorcluster)  [unwired: 1 in, 1 out]
                        }
                      }
                    }
                    frame True {
                      n215 = local read "ABORT"() -> (w828:bool)
                    }
                  }
                  n216 = Or(x=w796, y=w795) -> (x .or. y?=w797:bool)
                }
                n217 = node-c288 ("Output Node")(w226) -> (w225:errorcluster)
                n218 = local read "Save data"() -> (w175:bool)
                n219 = case shown="True" w175 {
                  tunnel: w223 -> [w230 w233]
                  tunnel: w222 -> [_ w232]
                  tunnel: [w230 w231] -> w211
                  frame False {
                  }
                  frame True {
                    n220 = Close File(refnum=w232, error in=w233) -> (error out=w231:errorcluster)  [unwired: 1 out]
                  }
                }
                n221 = node-c288 ("Output Node")(w228) -> (w224:errorcluster)
                n222 = RT FIFO Delete(0:w202, 2:TRUE ("force destroy? (F)"), 3:w204) -> (11:w203:errorcluster)
                n223 = node-c288(w214) -> (w210:errorcluster)
                n224 = local read "Water duration (uS)"() -> (w161:u32)
                n225 = local read "Lick threshold (V)"() -> (w162:fxp<+,32,16>)
                n226 = local read "Pulse delay"() -> (w153:sgl)
                n227 = RT FIFO Delete(0:w200, 2:TRUE ("force destroy? (F)"), 3:w199) -> (11:w198:errorcluster)
                n228 = node-c288("State machine cycle (uS)") -> (w217:T3)  [unwired: 3 in]
                n229 = Multiply(x=w153, y=sgl 1000.0) -> (x*y=w151:sgl)
                n230 = local read "VS threshold (V)"() -> (w163:fxp<+,32,16>)
                n231 = local read "Water refractory period (uS)"() -> (w159:u32)
                n232 = local read "Pulse period (ms)"() -> (w150:sgl)
                n233 = local read "Shock refractory period (uS)"() -> (w160:u32)
                n234 = Multiply(x=w150, y=sgl 1000.0) -> (x*y=w148:sgl)
                n235 = timed-loop {
                  timing: w217 -> [_]
                  timing-out: [_] -> w216
                  shift-right: [w439] -> _
                  shift-left: w158 -> [w452]
                  shift-right: [w441] -> _
                  shift-left: 1 -> [w453]
                  shift-right: [w438] -> _
                  shift-left: w158 -> [w447]
                  tunnel: w179 -> [w484]
                  shift-right: [w483] -> w206
                  shift-left: w178 -> [w482]
                  shift-right: [w442] -> _
                  shift-left: w201 -> [w454]
                  tunnel: w184 -> [w479]
                  shift-right: [w477] -> w197
                  shift-left: w183 -> [w478]
                  shift-right: [w480] -> _
                  shift-left: sgl[] [] ("array type (2D Dbl)") -> [w485]
                  tunnel: w144 -> [w470]
                  tunnel: [w463] -> w173
                  tunnel: w140 -> [w461]
                  tunnel: [w458] -> w171
                  tunnel: "VS filter period (uS)" -> [w423]
                  tunnel: w163 -> [w424]
                  tunnel: w162 -> [w456]
                  tunnel: w161 -> [w449]
                  tunnel: w160 -> [w443]
                  tunnel: w148 -> [w444]
                  tunnel: w159 -> [w446]
                  shift-right: [w437] -> _
                  shift-left: w158 -> [w451]
                  tunnel: w157 -> [w422]
                  tunnel: w151 -> [w410]
                  tunnel: w142 -> [w409]
                  tunnel: [w406] -> w145
                  shift-right: [w464] -> w174
                  shift-left: w143 -> [w469]
                  shift-right: [w407] -> w146
                  shift-left: w141 -> [w408]
                  shift-right: [w459] -> w170
                  shift-left: w139 -> [w460]
                  stop <- w471 stop-if-true
                  w435 = T1."Idle"
                  # "Ephys Trigger"
                  # "Pool 100 cycles"
                  # "ADD TRIAL #, Start and end of trial"
                  n236 = node-c288() -> (→"Actual cycle period (uS)":i64)  [unwired: 1 in, 1 out]
                  n237 = local read "Lick reward"() -> (w489:bool)
                  n238 = local read "Reward period (uS)"() -> (w450:u32)
                  n239 = shared-variable "My Computer\\Network variables.lvlib\\x degree out"() -> (w411:dbl)  [unwired: 1 in, 1 out]
                  "x degree out" <- w411
                  n240 = call-poly <vilib>:"DAQmx Read.vi"("task/channels in"=w470, "timeout"=0.1, "error in"=w469) -> ("task out"=w463:refnum<k21>, "data"=w466:dbl[], "error out"=w464:errorcluster)  [unwired: 10 in]
                  n241 = call "Tick Count"() -> ("Tick Count(uSec)"=w497:u32)
                  n242 = Index Array(array=w466, index #1=0 ("index"), index #2=1 ("index"), index #3=2 ("index"), index #4=3 ("index"), index #5=4 ("index")) -> (element #1=w457:dbl, element #2=w465:dbl, element #3=w425:dbl, element #4=w421:dbl, element #5=w428:dbl)
                  n243 = feedback #1(FALSE) -> (w492:bool)
                  n244 = feedback-in #1(w489) -> ()
                  n245 = feedback #2(w497) -> (w498:u32)
                  n246 = feedback-in #2(w497) -> ()
                  n247 = local read "Trial timeout (uS)"() -> (w445:u32)
                  n248 = Greater?(x=w489, y=w492) -> (0:w490:bool)
                  n249 = Subtract(x=w497, y=w498) -> (x-y=w496:u32)
                  n250 = call "vs digital filter3.vi"("filter period(uSec)"=w423, "vs threshold"=w424, "input"=w425) -> ("output"=w418:bool)  [unwired: 3 in]
                  n251 = To Unsigned Quad Integer(1:w496) -> (0:w495:u64)
                  n252 = Greater?(x=w465, y=w456) -> (0:w417:bool)
                  n253 = feedback #3(u64 0) -> (w494:u64)
                  n254 = Add(x=w495, y=w494) -> (x+y=w448:u64)
                  n255 = Divide(x=w448, y=u64 1000) -> (x/y=w487:dbl)
                  n256 = feedback-in #3(w448) -> ()
                  n257 = call "vs digital filter.vi"("filter period(uSec)"=w423, "vs threshold"=w424, "input"=w457) -> ("output"=w420:bool)  [unwired: 3 in]
                  n258 = feedback #4(w435) -> (w499:T1)
                  n259 = Select(t=T1."Lick reward", s=w490, f=w499) -> (s? t:f=w431:T1)
                  n260 = feedback #5(w435) -> (w436:T1)
                  n261 = local read "ABORT"() -> (w471:bool)
                  n262 = Build Array(w487, w453, w431, w421) -> (w414:dbl[])
                  n263 = To Single Precision Float(number=w414) -> (single precision float=w415:sgl[])
                  n264 = local read "Manually give water"() -> (w488:bool)
                  n265 = shared-variable "My Computer\\Network variables.lvlib\\stop - network"() -> (w500:bool)  [unwired: 1 in, 1 out]
                  n266 = call "vs digital filter2.vi"("filter period(uSec)"=w423, "vs threshold"=w424, "input"=w428) -> ("output"=w419:bool)  [unwired: 3 in]
                  n267 = feedback #6(0.0 ("Double")) -> (w403:dbl)
                  n268 = case shown="\"VS\"" w431 {
                    selector: w431 -> [w515 w525 w539 w576 w587 w611 _ w635 w666 w694 _ w720 w729 w757]
                    tunnel: w454 -> [w516 w533 w558 w580 w604 w616 w628 w648 w670 w696 w712 w722 w741 w760]
                    tunnel: w453 -> [w512 w532 w557 w579 w602 w615 w627 w646 w669 w695 w711 w721 w740 w762]
                    tunnel: w417 -> [_ _ _ _ w590 _ _ _ _ _ _ _ _ w756]
                    tunnel: w452 -> [w511 w531 w556 w578 w594 w614 w624 w645 w656 w692 w709 w719 w735 w755]
                    tunnel: w451 -> [w510 w530 w554 w573 w600 w613 w623 w644 w662 w691 w708 w718 w738 w754]
                    tunnel: w450 -> [_ _ _ _ w598 _ _ _ _ _ _ _ _ _]
                    tunnel: w449 -> [_ _ _ _ _ _ _ w643 _ _ _ _ _ w753]
                    tunnel: w448 -> [_ _ _ w570 w593 _ _ w638 w659 w685 _ _ w732 w749]
                    tunnel: w447 -> [w509 w529 w555 w577 w599 w612 w622 w640 w661 w690 w698 w717 w737 w750]
                    tunnel: w410 -> [_ _ _ w571 _ _ _ _ _ _ _ _ _ _]
                    tunnel: w446 -> [_ _ _ _ _ _ _ _ _ _ _ _ _ _]
                    tunnel: w445 -> [_ _ _ _ _ _ _ _ w665 _ _ _ w733 _]
                    tunnel: w444 -> [_ _ _ _ _ _ _ _ _ w687 _ _ _ _]
                    tunnel: w443 -> [_ _ _ _ _ _ _ _ _ _ _ _ _ _]
                    tunnel: [w516 w533 w558 w580 w604 w616 w628 w647 w670 w696 w712 w722 w741 w761] -> w442
                    tunnel: [w512 w532 w557 w579 w602 w615 w626 w646 w669 w695 w711 w721 w740 w762] -> w441
                    tunnel: [w513 w528 w552 w563 w603 w611 T1."Idle" w637 w668 w678 w710 w720 w731 w758] -> w432
                    tunnel: [FALSE w521 w534 w559 w581 w607 w617 TRUE FALSE FALSE w697 w713 w723 w756] -> w440
                    tunnel: [w511 w531 w556 w578 w592 w614 w624 w645 w656 w692 w709 w719 w728 w755] -> w439
                    tunnel: [w509 w529 w555 w577 w599 w612 w622 w639 w660 w682 w698 w717 w737 w747] -> w438
                    tunnel: [w510 w530 w554 w568 w600 w613 w623 w644 w662 w691 w708 w718 w738 w754] -> w437
                    tunnel: w436 -> [_ _ _ w575 w597 _ _ w650 w667 w693 _ _ w739 w759]
                    tunnel: w420 -> [_ w527 w551 w565 _ _ _ _ _ w681 w707 _ _ _]
                    tunnel: w403 -> [w507 _ w549 _ w584 w608 _ _ _ _ _ w714 _ _]
                    tunnel: [w507 0.0 ("Double") w548 w562 w584 w608 w618 w630 w652 w672 w699 w714 w724 w743] -> w405
                    tunnel: w411 -> [_ _ w548 w562 _ _ w618 w630 w652 w672 w699 _ w724 w743]
                    tunnel: w409 -> [w505 w522 w535 w560 w582 w609 w619 w631 w653 w676 w705 w715 w726 w745]
                    tunnel: w408 -> [w506 w523 w536 w561 w583 w610 w620 w632 w654 w677 w704 w716 w725 w744]
                    tunnel: [w503 w522 w535 w560 w582 w609 w619 w631 w653 w675 w702 w715 w726 w745] -> w406
                    tunnel: [w502 w523 w536 w561 w583 w610 w620 w632 w654 w674 w701 w716 w725 w744] -> w407
                    tunnel: [FALSE w521 w534 w559 w581 w607 w617 FALSE FALSE TRUE w697 w713 w723 FALSE] -> w402
                    frame "Idle", Default {
                      n269 = local read "Start one trial"() -> (w514:bool)
                      n270 = call-poly <vilib>:"DAQmx Write.vi"("task/channels in"=w505, "data"=0.0, "error in"=w506) -> ("task out"=w503:refnum<k21>, "error out"=w502:errorcluster)  [unwired: 10 in, 1 out]
                      n271 = case shown="True" w514 {
                        tunnel: w515 -> [w517 _]
                        tunnel: [w517 w518] -> w513
                        frame False {
                        }
                        frame True {
                          n272 = stacked-sequence {
                            tunnel: [T1."Before VS" _] -> w518
                            frame #0 {
                            }
                            frame #1 {
                              w520 = FALSE
                              n273 = local write "Start one trial"(w520) -> ()
                              n274 = local write "Trial Done"(w520) -> ()
                            }
                          }
                        }
                      }
                    }
                    frame "Before VS" {
                      w521 = FALSE
                      n275 = Select(t=T1."VS", s=w527, f=w525) -> (s? t:f=w528:T1)
                    }
                    frame "VS" {
                      w534 = FALSE
                      n276 = local read "Saccade min degrees per 3 frames"() -> (w544:dbl)
                      n277 = local read "Saccade max degrees per 3 frames"() -> (w545:dbl)
                      n278 = Subtract(x=w548, y=w549) -> (x-y=w547:dbl)
                      n279 = Absolute Value(x=w547) -> (abs(x)=w546:dbl)
                      n280 = Greater Or Equal?(x=w546, y=w544) -> (x >= y?=w543:bool)
                      n281 = Less Or Equal?(x=w546, y=w545) -> (x <= y?=w542:bool)
                      n282 = local read "LED?"() -> (w550:bool)
                      n283 = And(x=w543, y=w542) -> (x .and. y?=w541:bool)
                      n284 = And(x=w550, y=w541) -> (x .and. y?=w540:bool)
                      n285 = Select(t=T1."VS2", s=w540, f=w539) -> (s? t:f=w538:T1)
                      n286 = Select(t=w538, s=w551, f=T1."After VS") -> (s? t:f=w552:T1)
                    }
                    frame "VS2" {
                      w559 = FALSE
                      # "Delay before LED!"
                      # "Punish=LED!!"
                      n287 = Equal?(x=w576, y=w575) -> (x = y?=w574:bool)
                      n288 = Add(x=w570, y=w571) -> (x+y=w572:sgl)
                      n289 = Select(t=w573, s=w574, f=w572) -> (s? t:f=w568:sgl)
                      n290 = Greater?(x=w568, y=w570) -> (0:w569:bool)
                      n291 = Select(t=w576, s=w569, f=T1."Punish") -> (s? t:f=w564:T1)
                      n292 = Select(t=w564, s=w565, f=T1."After VS") -> (s? t:f=w563:T1)
                    }
                    frame "After VS" {
                      w581 = FALSE
                      n293 = Equal?(x=w587, y=w597) -> (x = y?=w595:bool)
                      n294 = Add(x=w598, y=w593) -> (x+y=w596:u64)
                      n295 = Select(t=w594, s=w595, f=w596) -> (s? t:f=w592:u64)
                      n296 = Greater?(x=w592, y=w593) -> (0:w591:bool)
                      n297 = Select(t=T1."Reward", s=w590, f=w587) -> (s? t:f=w588:T1)
                      n298 = Select(t=w588, s=w591, f=T1."Cycle End") -> (s? t:f=w601:T1)
                      n299 = case shown="True" "Automatic reward" {
                        tunnel: [w605 T1."Reward"] -> w603
                        tunnel: w601 -> [w605 _]
                        frame False {
                        }
                        frame True {
                        }
                      }
                    }
                    frame "Wait for lever press" {
                      w607 = FALSE
                    }
                    frame "Cycle End" {
                      w617 = FALSE
                      n300 = Increment(x=w627) -> (x+1=w626:i32)
                      n301 = local write "Trial Done"(TRUE) -> ()
                    }
                    frame "Reward" {
                      n302 = Add(x=w643, y=w638) -> (x+y=w642:u64)
                      n303 = Increment(x=w648) -> (x+1=w649:i32)
                      n304 = Equal?(x=w635, y=w650) -> (x = y?=w641:bool)
                      n305 = Select(t=w640, s=w641, f=w642) -> (s? t:f=w639:sgl)
                      n306 = Select(t=w648, s=w641, f=w649) -> (s? t:f=w647:i32)
                      "# of rewards" <- w647
                      n307 = Greater?(x=w639, y=w638) -> (0:w636:bool)
                      n308 = Select(t=w635, s=w636, f=T1."Cycle End") -> (s? t:f=w637:T1)
                    }
                    frame "Reward Refractory" {
                      n309 = Equal?(x=w666, y=w667) -> (x = y?=w663:bool)
                      n310 = Add(x=w659, y=w665) -> (x+y=w664:u64)
                      n311 = Select(t=w661, s=w663, f=w664) -> (s? t:f=w660:sgl)
                      n312 = Greater?(x=w660, y=w659) -> (0:w658:bool)
                      n313 = Select(t=w666, s=w658, f=T1."Cycle End") -> (s? t:f=w668:T1)
                    }
                    frame "Punish" {
                      # "=LED!!"
                      n314 = Equal?(x=w694, y=w693) -> (x = y?=w689:bool)
                      n315 = local read "Pulse amp 0"() -> (w673:sgl)
                      n316 = Add(x=w685, y=w687) -> (x+y=w688:sgl)
                      n317 = Select(t=w690, s=w689, f=w688) -> (s? t:f=w682:sgl)
                      n318 = call-poly <vilib>:"DAQmx Write.vi"("task/channels in"=w676, "data"=w673, "error in"=w677) -> ("task out"=w675:refnum<k21>, "error out"=w674:errorcluster)  [unwired: 10 in, 1 out]
                      n319 = Greater?(x=w682, y=w685) -> (0:w686:bool)
                      n320 = Select(t=w694, s=w686, f=T1."Punish Refractory") -> (s? t:f=w679:T1)
                      n321 = Select(t=w679, s=w681, f=T1."Punish Refractory") -> (s? t:f=w678:T1)
                    }
                    frame "Punish Refractory" {
                      w697 = FALSE
                      # "Possibly code LED refractory period"
                      # "STOP LED HERE!"
                      n322 = call-poly <vilib>:"DAQmx Write.vi"("task/channels in"=w705, "data"=0.0, "error in"=w704) -> ("task out"=w702:refnum<k21>, "error out"=w701:errorcluster)  [unwired: 10 in, 1 out]
                      n323 = Select(t=T1."VS", s=w707, f=T1."After VS") -> (s? t:f=w710:T1)
                    }
                    frame "Exit" {
                      w713 = FALSE
                    }
                    frame "Timeout" {
                      w723 = FALSE
                      # "Can be used for pre-VS state for suppressing LED"
                      n324 = Equal?(x=w729, y=w739) -> (x = y?=w736:bool)
                      n325 = Add(x=w732, y=w733) -> (x+y=w734:u64)
                      n326 = Select(t=w735, s=w736, f=w734) -> (s? t:f=w728:u64)
                      n327 = Greater?(x=w728, y=w732) -> (0:w730:bool)
                      n328 = Select(t=w729, s=w730, f=T1."Cycle End") -> (s? t:f=w731:T1)
                    }
                    frame "Lick reward" {
                      n329 = Equal?(x=w757, y=w759) -> (x = y?=w752:bool)
                      n330 = Add(x=w753, y=w749) -> (x+y=w751:u64)
                      n331 = Select(t=w750, s=w752, f=w751) -> (s? t:f=w747:sgl)
                      n332 = Greater?(x=w747, y=w749) -> (0:w748:bool)
                      n333 = case shown="True" w756 {
                        tunnel: [w763 w765] -> w761
                        tunnel: w760 -> [w763 w764]
                        frame False {
                        }
                        frame True {
                          n334 = Increment(x=w764) -> (x+1=w765:i32)
                        }
                      }
                      n335 = Select(t=w757, s=w748, f=T1."Reward Refractory") -> (s? t:f=w758:T1)
                    }
                  }
                  n336 = Select(t=T1."Exit", s=w500, f=w432) -> (s? t:f=w455:T1)
                  n337 = feedback-in #4(w455) -> ()
                  n338 = feedback-in #5(w455) -> ()
                  n339 = Or(x=w488, y=w440) -> (x .or. y?=w416:bool)
                  n340 = Build Array(w418, w402, w416) -> (w474:bool[])
                  n341 = Boolean Array To Number(Boolean array=w474) -> (number=w412:u32)
                  n342 = To Single Precision Float(number=w412) -> (single precision float=w413:sgl)
                  n343 = Build Array (concatenate)(w415, w413) -> (w473:sgl[])
                  n344 = Build Array (concatenate)(w485, w473) -> (w481:sgl[])
                  n345 = Array Size(array=w481) -> (size(s)=w476:i32)
                  n346 = Equal?(x=w476, y=w422) -> (x = y?=w475:bool)
                  n347 = case shown="True" w475 {
                    tunnel: w484 -> [_ w778]
                    tunnel: [w768 w777] -> w483
                    tunnel: w482 -> [w768 w775]
                    tunnel: w481 -> [w767 w772]
                    tunnel: [w767 sgl[] [] ("array type (2D Dbl)")] -> w480
                    tunnel: w479 -> [_ w771]
                    tunnel: w478 -> [w766 w770]
                    tunnel: [w766 w769] -> w477
                    frame False {
                    }
                    frame True {
                      n348 = RT FIFO Write(0:w778, 1:w772, 2:10 ("timeout in ms (0)"), 3:w775) -> (11:w777:errorcluster)  [unwired: 1 in, 3 out]
                      n349 = RT FIFO Write(0:w771, 1:w772, 2:10 ("timeout in ms (0)"), 3:w770) -> (11:w769:errorcluster)  [unwired: 1 in, 3 out]
                    }
                  }
                  n350 = Build Array(w416, w419, w418) -> (w462:bool[])
                  n351 = feedback-in #6(w405) -> ()
                  n352 = node-c288() -> ()  [unwired: 3 in, 1 out]
                  n353 = call-poly <vilib>:"DAQmx Write.vi"("task/channels in"=w461, "data"=w462, "error in"=w460) -> ("task out"=w458:refnum<k21>, "error out"=w459:errorcluster)  [unwired: 10 in, 1 out]
                }
                n354 = node-c288(w216) -> (w209:errorcluster)
                n355 = call <vilib>:"DAQmx Stop Task.vi"("task/channels in"=w145, "error in"=w146) -> ("error out"=w147:errorcluster)  [unwired: 12 in, 1 out]
                n356 = call <vilib>:"DAQmx Stop Task.vi"("task/channels in"=w173, "error in"=w174) -> ("error out"=w172:errorcluster)  [unwired: 12 in, 1 out]
                n357 = Merge Errors(w203, w206, w198, w197) -> (w205:errorcluster)
                n358 = Build Array(w165, w165, w165) -> (w167:bool[])
                n359 = call-poly <vilib>:"DAQmx Write.vi"("task/channels in"=w171, "data"=w167, "error in"=w170) -> ("task out"=w169:refnum<k21>, "error out"=w168:errorcluster)  [unwired: 10 in, 1 out]
                n360 = call <vilib>:"DAQmx Stop Task.vi"("task/channels in"=w169, "error in"=w168) -> ("error out"=w187:errorcluster)  [unwired: 12 in, 1 out]
                n361 = Merge Errors(w172, w187, w147) -> (w207:errorcluster)
                n362 = stacked-sequence {
                  tunnel: w224 -> [w794]
                  tunnel: w225 -> [w793]
                  tunnel: w211 -> [w791]
                  tunnel: w210 -> [w790]
                  tunnel: w209 -> [w789]
                  tunnel: w207 -> [w788]
                  tunnel: w205 -> [w787]
                  frame #0 {
                    n363 = Merge Errors(w789, w790, w794, w793, w791, w788, w787) -> (w792:errorcluster)
                    "error out" <- w792
                    n364 = call <vilib>:"Simple Error Handler.vi"("error in (no error)"=w792) -> ()  [unwired: 4 in, 5 out]
                  }
                }
              }
            }
          }
          frame #2 {
            n365 = Wait (ms)(milliseconds to wait=u32 50) -> ()  [unwired: 1 out]
          }
        }
      }
      n366 = UDP Close(connection ID=w2, 8:w3) -> (error out=w1:errorcluster)  [unwired: 1 out]
      n367 = call <vilib>:"Simple Error Handler.vi"("error in (no error)"=w1) -> ()  [unwired: 4 in, 5 out]
    }
    frame #1 {
      w1029 = FALSE
      n368 = local write "Busy"(w1029) -> ()
      n369 = local write "ABORT"(w1029) -> ()
      n370 = local write "Initial data received"(w1029) -> ()
      n371 = local write "Stop state"(w1029) -> ()
    }
  }
